vi "UE9 eDI CR performance tester.vi"() -> (0 "error out":errorcluster)   [LabVIEW 2021]
panel:
  in  "ConnectionType":u16(ring) items=["LJ_ctUSB", "LJ_ctETHERNET"]
  out "Avg ms Per Iteration":dbl format="%.2f"
  out "Total ms":u32
  out "Min Interval":u32
  out "Max Interval":u32
  out "Intervals":u32[](array[numeric])
  in  "Number of Iterations":u32=1000
  in  "stop":bool
  in  "Interval (ms)":u32
  in  "FirstFound":bool=TRUE
  in  "Address":string="192.168.1.209"
  out "Error Message":string
  # "Specify an IP address for Ethernet, or Local ID\nfor USB.  If FirstFound is selected, Local ID is\nignored for USB."
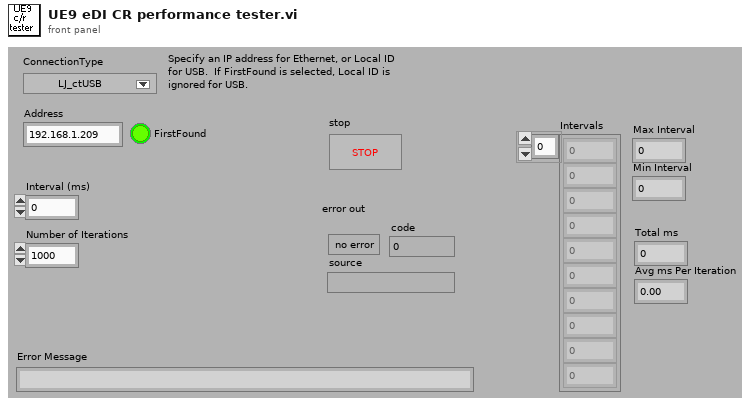
[diagram p1: front panel]
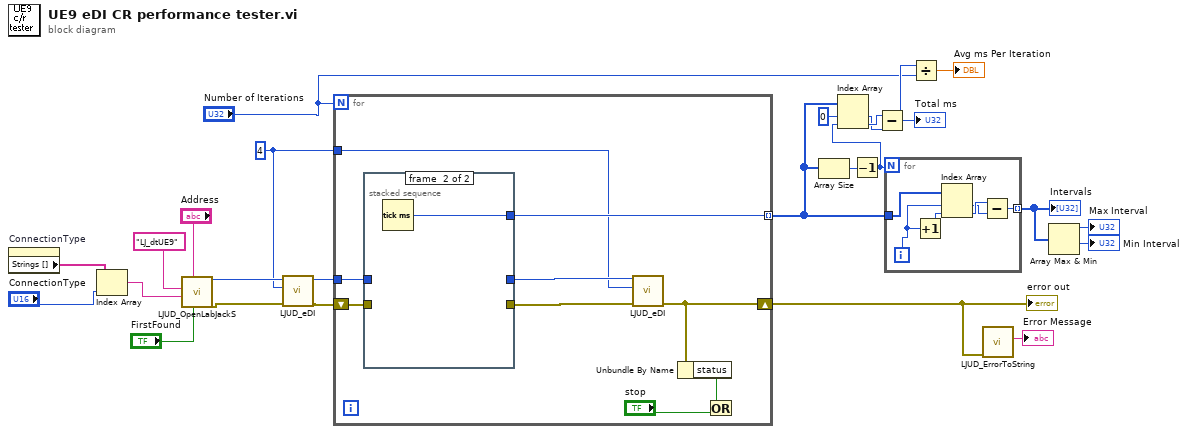
[diagram p0: block diagram]
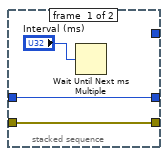
[diagram p2: hidden frame]
diagram:
  w1 = 4 ("Channel")
  n1 = property on="ConnectionType" class="Ring (strict)"() -> ("Strings []"=w8:string[])  [unwired: 2 in, 2 out]
  n2 = Index Array(array=w8, index="ConnectionType") -> (element=w6:string)
  n3 = call "LJUD_OpenLabJackS.vi"("FirstFound"="FirstFound", "Address"="Address", "ConnectionType"=w6, "DeviceType"="LJ_dtUE9") -> ("error out"=w3:errorcluster, "Handle"=w2:i32)  [unwired: 5 in, 1 out]
  n4 = call "LJUD_eDI.vi"("error in"=w3, "Channel"=w1, "Handle In"=w2) -> ("error out"=w4:errorcluster, "Handle Out"=w5:i32)  [unwired: 6 in, 1 out]
  n5 = for {
    N: "Number of Iterations" -> [_]
    tunnel: w5 -> [w31]
    shift-right: [w33] -> w21
    shift-left: w4 -> [w30]
    tunnel: [w27] -> w16 mode=indexing
    tunnel: w1 -> [w26]
    n6 = stacked-sequence {
      tunnel: w31 -> [w35 _]
      tunnel: w30 -> [w36 _]
      tunnel: [w36 _] -> w29
      tunnel: [w35 _] -> w28
      tunnel: [_ w38] -> w27
      frame #0 {
        n7 = Wait Until Next ms Multiple(millisecond multiple="Interval (ms)") -> ()  [unwired: 1 out]
      }
      frame #1 {
        n8 = Tick Count (ms)() -> (millisecond timer value=w38:u32)
      }
    }
    n9 = call "LJUD_eDI.vi"("error in"=w29, "Channel"=w26, "Handle In"=w28) -> ("error out"=w33:errorcluster)  [unwired: 6 in, 2 out]
    n10 = Unbundle By Name(w33) -> ("status"=w34:bool)
    n11 = Or(x=w34, y="stop") -> ()  [unwired: 1 out]
  }
  "error out" <- w21
  n12 = Array Size(array=w16) -> (size(s)=w20:i32)
  n13 = Decrement(x=w20) -> (x-1=w14:i32)
  n14 = Index Array(array=w16, index #1=0 ("Index"), index #2=w14) -> (element #1=w9:u32, element #2=w10:u32)
  n15 = Subtract(x=w10, y=w9) -> (x-y=w13:u32)
  "Total ms" <- w13
  n16 = for {
    N: w14 -> [_]
    tunnel: w16 -> [w44]
    tunnel: [w41] -> w19 mode=indexing
    i -> [w42]
    n17 = Increment(x=w42) -> (x+1=w43:i32)
    n18 = Index Array(array=w44, index #1=w42, index #2=w43) -> (element #1=w39:u32, element #2=w40:u32)
    n19 = Subtract(x=w40, y=w39) -> (x-y=w41:u32)
  }
  "Intervals" <- w19
  n20 = Divide(x=w13, y="Number of Iterations") -> (x/y=→"Avg ms Per Iteration":dbl)
  n21 = call "LJUD_ErrorToString.vi"("error in"=w21) -> ("String"=→"Error Message":string)  [unwired: 10 in]
  n22 = Array Max & Min(array=w19) -> (max value=→"Max Interval":u32, min value=→"Min Interval":u32)  [unwired: 2 out]
